vi "Handle Data Request.vi"(6 "Promise":refnum<class "Promise.lvclass">, 8 "error in (no error)":errorcluster, 10 "Data Request":T1, 11 "Historian Module in":refnum<class "Historian Module.lvclass">) -> (0 "error out":errorcluster, 3 "Historian Module out":refnum<class "Historian Module.lvclass">)   [LabVIEW 2020, in "VolatusHistorian.lvlib" / "Historian Module.lvclass"]
uses:
  Historian Module.lvclass
  Data Request.ctl
  Time Format.ctl
  lv-promises/Promises/Promise/Promise.lvclass
  Historian Module.lvclass/Historian Module.ctl
  Needed Group Data.ctl
  VolatusHistorian.lvlib
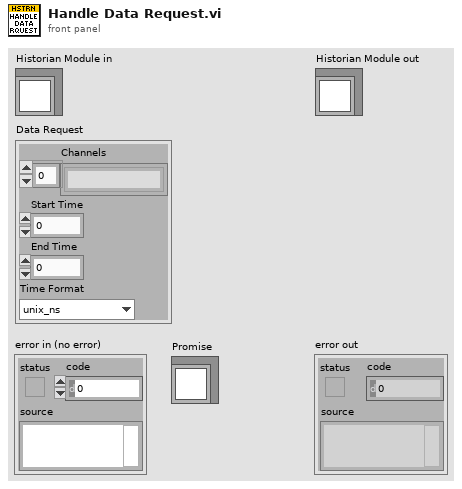
[diagram p1: front panel]
types:
  T1 = typedef "VolatusHistorian.lvlib/Data Request.ctl" = cluster{"Channels":string[], "Start Time":dbl, "End Time":dbl, "Time Format":T2}
  T2 = typedef "VolatusHistorian.lvlib/Time Format.ctl" = enum16{"unix_ns", "lv"}
  T3 = typedef "VolatusHistorian.lvlib/Historian Module.lvclass/Historian Role.ctl" = enum16{"Primary", "Local"}
  T4 = typedef "VolatusHistorian.lvlib/Historian Module.lvclass/Needed Group Data.ctl" = cluster{"Group":string, "Channels":string[], "Start":dbl, "End":dbl}
  T5 = typedef "VolatusHistorian.lvlib/Historian Module.lvclass/Grouped Channels.ctl" = map{string, string[]}
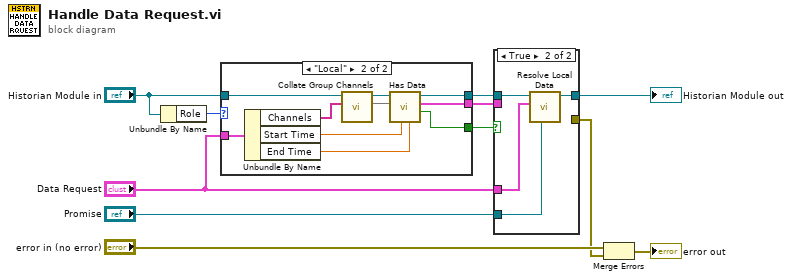
[diagram p0: block diagram]
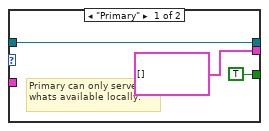
[diagram p2: hidden frame]
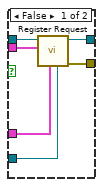
[diagram p3: hidden frame]
diagram:
  n1 = Unbundle By Name("Historian Module in") -> ("Role"=w3:T3)
  n2 = case shown="\"Local\"" w3 {
    tunnel: [TRUE ("Has Data") w19] -> w10
    tunnel: [T4[] [] ("Needed Data") w18] -> w9
    tunnel: [w14 w17] -> w8
    tunnel: "Data Request" -> [_ w16]
    tunnel: "Historian Module in" -> [w14 w15]
    frame "Primary" {
      # "Primary can only serve whats available locally."
    }
    frame "Local" {
      n3 = Unbundle By Name(w16) -> ("Channels"=w24:string[], "Start Time"=w21:dbl, "End Time"=w20:dbl)
      n4 = call "Collate Group Channels.vi"("Channel Names"=w24, "Historian Module in"=w15) -> ("Grouped Channels"=w22:T5, "Historian Module out"=w23:refnum<class "Historian Module.lvclass">)  [unwired: 7 in, 1 out]
      n5 = call "Has Data.vi"("End"=w20, "Start"=w21, "Grouped Channels"=w22, "Historian Module in"=w23) -> ("Has Data"=w19:bool, "Needed Data"=w18:T4[], "Historian Module out"=w17:refnum<class "Historian Module.lvclass">)  [unwired: 5 in]
    }
  }
  n6 = case shown="True" w10 {
    tunnel: w9 -> [w29 _]
    tunnel: w8 -> [w30 w34]
    tunnel: "Data Request" -> [w28 w33]
    tunnel: "Promise" -> [w27 w32]
    tunnel: [w26 w31] -> w5
    tunnel: [w25 _] -> w1
    frame False {
      n7 = call "Register Request.vi"("Promise"=w27, "Data Request"=w28, "Needed Data"=w29, "Historian Module in"=w30) -> ("error out"=w25:errorcluster, "Historian Module out"=w26:refnum<class "Historian Module.lvclass">)  [unwired: 6 in]
    }
    frame True {
      n8 = call "Resolve Local Data.vi"("Promise"=w32, "Data Request"=w33, "Historian Module in"=w34) -> ("Historian Module out"=w31:refnum<class "Historian Module.lvclass">)  [unwired: 7 in, 1 out]
    }
  }
  "Historian Module out" <- w5
  n9 = Merge Errors("error in (no error)", w1) -> (→"error out":errorcluster)
